vi "Parse_error_array.vi"(11 "Error array":string[][](array[string])) -> (3 "Error string":string)   [LabVIEW 2017, in "labview-standard-library.lvlib"]
uses:
  labview-standard-library.lvlib
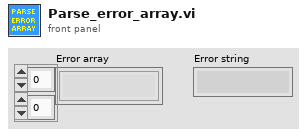
[diagram p1: front panel]
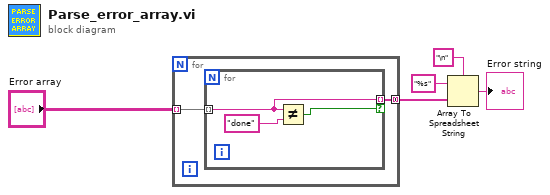
[diagram p0: block diagram]
diagram:
  n1 = for {
    tunnel: "Error array" -> [w7] mode=indexing
    tunnel: [w6] -> w3 mode=concatenating
    n2 = for {
      tunnel: w7 -> [w9] mode=indexing
      tunnel: [w9] -> w6 mode=indexing if=w8
      n3 = Not Equal?(x=w9, y="done") -> (x != y?=w8:bool)
    }
  }
  n4 = Array To Spreadsheet String(delimiter (Tab)="\n", array=w3, 3:"%s" ("format string")) -> (spreadsheet string=→"Error string":string)
